vi "Excel_Color_to_RGB.vi"(0 "excel color table index":i32) -> (1 "R":u8, 2 "G":u8, 3 "B":u8)   [LabVIEW 2017, in "NI_ReportGenerationToolkit.lvlib"]
uses:
  <vilib>/addons/_office/NI_ReportGenerationToolkit.lvlib
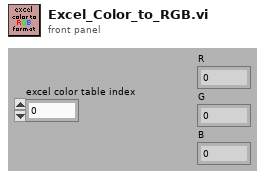
[diagram p1: front panel]
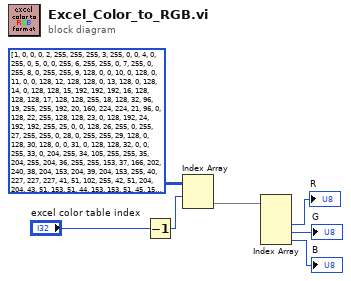
[diagram p0: block diagram]
diagram:
  n1 = Decrement(x="excel color table index") -> (x-1=w5:i32)
  n2 = Index Array(array=i32[][] [[1, 0, 0, 0], [2, 255, 255, 255], [3, 255, 0, 0], [4, 0, 255, 0], [5, 0, 0, 255], [6, 255, 255, 0], [7, 255, 0, 255], [8, 0, 255, 255], [9, 128, 0, 0], [10, 0, 128, 0], [11, 0, 0, 128], [12, 128, 128, 0], [13, 128, 0, 128], [14, 0, 128, 128], [15, 192, 192, 192], [16, 128, 128, 128], [17, 128, 128, 255], [18, 128, 32, 96], [19, 255, 255, 192], [20, 160, 224, 224], [21, 96, 0, 128], [22, 255, 128, 128], [23, 0, 128, 192], [24, 192, 192, 255], [25, 0, 0, 128], [26, 255, 0, 255], [27, 255, 255, 0], [28, 0, 255, 255], [29, 128, 0, 128], [30, 128, 0, 0], [31, 0, 128, 128], [32, 0, 0, 255], [33, 0, 204, 255], [34, 105, 255, 255], [35, 204, 255, 204], [36, 255, 255, 153], [37, 166, 202, 240], [38, 204, 153, 204], [39, 204, 153, 255], [40, 227, 227, 227], [41, 51, 102, 255], [42, 51, 204, 204], [43, 51, 153, 51], [44, 153, 153, 51], [45, 153, 102, 51], [46, 153, 102, 102], [47, 102, 102, 153], [48, 150, 150, 150], [49, 51, 51, 204], [50, 51, 102, 102], [51, 0, 51, 0], [52, 51, 51, 0], [53, 102, 51, 0], [54, 153, 51, 102], [55, 51, 51, 153], [56, 66, 66, 66]] ("data"), index (row)=w5) -> (element=w4:i32[])  [unwired: 1 in]
  n3 = Index Array(array=w4) -> (element #2=→"R":i32, element #3=→"G":i32, element #4=→"B":i32)  [unwired: 4 in, 1 out]
